vi "Set Message Stream.vi"(10 "Message Stream.lvclass":refnum<class "Message Stream.lvclass">, 11 "Study Actor in":refnum<class "Study Actor.lvclass">) -> (3 "Study Actor out":refnum<class "Study Actor.lvclass">)   [LabVIEW 2023, in "Study Actor.lvlib" / "Study Actor.lvclass"]
uses:
  Study Actor.lvclass
  <vilib>/ni/Actors/Network Endpoint Actors/Abstract Classes/Message Stream/Message Stream.lvclass
  Study Actor.lvclass/Study Actor.ctl
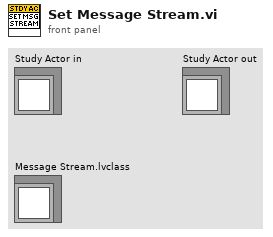
[diagram p1: front panel]
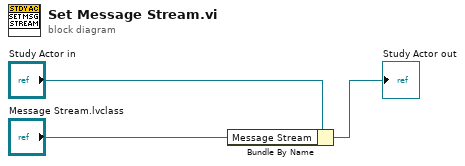
[diagram p0: block diagram]
diagram:
  n1 = Bundle By Name(cluster="Study Actor in", "Message Stream"="Message Stream.lvclass") -> (→"Study Actor out":refnum<class "Study Actor.lvclass">)
